vi "Get UI Details.vi"() -> ()   [LabVIEW 2021, in "AC_Audio ADC.lvlib"]
uses:
  AC_Audio ADC.lvlib
  <vilib>/MeasurementLink/MeasurementLink Measurement Server/Helpers/TypeDefs/User Interface Information.ctl
  <vilib>/MeasurementLink/MeasurementLink Measurement Server/MeasurementLink Measurement Server.lvlib
panel:
  out "error out":errorcluster
  in  "error in (no error)":errorcluster
  out "user interface details":T1[](array[typedef])
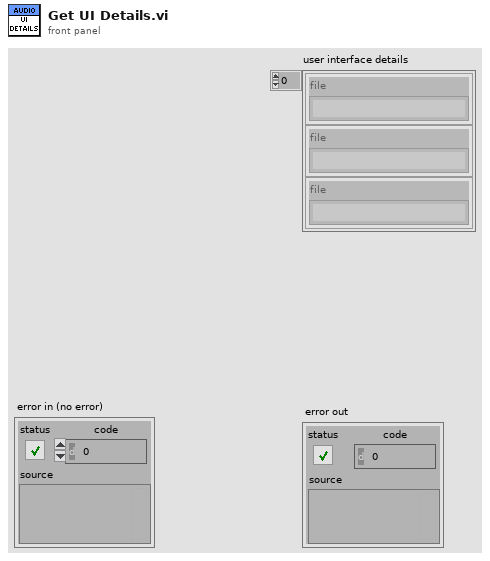
[diagram p1: front panel]
types:
  T1 = typedef "MeasurementLink Measurement Server.lvlib/User Interface Information.ctl" = cluster{"file":string}
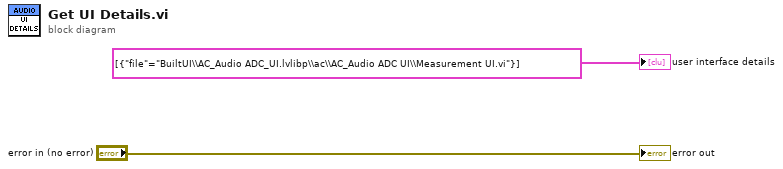
[diagram p0: block diagram]
diagram:
  "user interface details" <- T1[] [{"file"="BuiltUI\\AC_Audio ADC_UI.lvlibp\\ac\\AC_Audio ADC UI\\Measurement UI.vi"}] ("UI Details")
  "error out" <- "error in (no error)"
